vi "Close_Instr.vi"(8 "error in (no error)":errorcluster caption="entrée d'erreur (pas d'erreur)", 11 "Class Instrument Multimeter en entrée":refnum<class "Class Instrument Multimeter.lvclass">) -> (0 "error out":errorcluster caption="sortie d'erreur", 3 "Class Instrument Multimeter en sortie":refnum<class "Class Instrument Multimeter.lvclass">)   [LabVIEW 2020, in "Library Instrument & Equipement.lvlib" / "Library Instruments.lvlib" / "Class Instrument Multimeter.lvclass"]
uses:
  Class Instrument Multimeter.lvclass
  Class Instrument Multimeter.lvclass/Class Instrument Multimeter.ctl
  Multimeter/Multimeter (Default)/Class Multimeter (Default).lvclass
  Instrument (Default)/Class Instrument (Default).lvclass
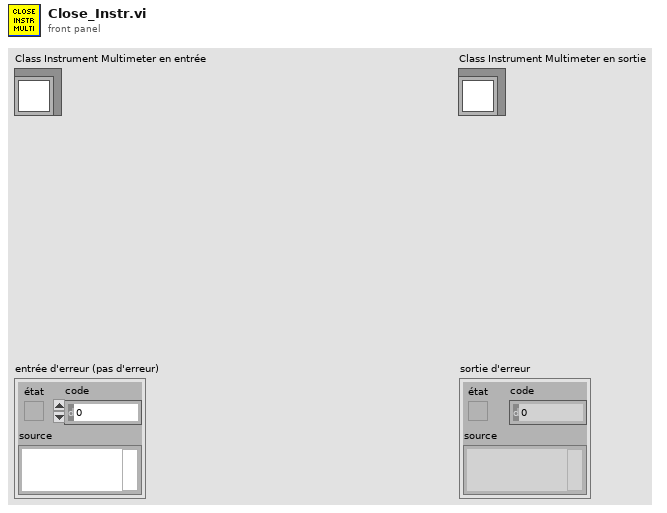
[diagram p1: front panel]
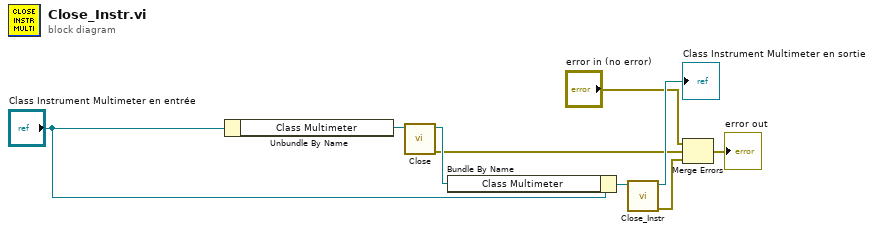
[diagram p0: block diagram]
diagram:
  n1 = Unbundle By Name("Class Instrument Multimeter en entrée") -> ("Class Multimeter"=w9:refnum<class "Class Multimeter (Default).lvclass">)
  n2 = call-dynamic "Close.vi"("Class Multimeter (Default) en entrée"=w9) -> ("error out"=w3:errorcluster, "Class Multimeter (Default) en sortie"=w7:refnum<class "Class Multimeter (Default).lvclass">)  [unwired: 9 in]
  n3 = Bundle By Name(cluster="Class Instrument Multimeter en entrée", "Class Multimeter"=w7) -> (w5:refnum<class "Class Instrument Multimeter.lvclass">)
  n4 = call-parent "Close_Instr.vi"("Class Instrument (Default) en entrée"=w5) -> ("error out"=w2:errorcluster, "Class Instrument (Default) en sortie"=→"Class Instrument Multimeter en sortie":refnum<class "Class Instrument Multimeter.lvclass">)  [unwired: 9 in]
  n5 = Merge Errors("error in (no error)", w3, w2) -> (→"error out":errorcluster)
